vi "Test Get Data.vi"() -> ()   [LabVIEW 2014]
uses:
  FPGA/Rate.ctl
  <vilib>/FPGAPlugInAG/sbRIO-9636/niLvFpga_Open_sbRIO-9636.vi
  <vilib>/Utility/error.llb/Error Cluster From Error Code.vi
  <vilib>/rvi/errors/niLvFpgaAdjustHostInterfaceError.vi
  <vilib>/rvi/interface/common/niFpgaWaitOnOcc.vi
  <vilib>/FPGAPlugInAG/sbRIO-9636/niLvFpga_Close_sbRIO-9636.vi
  <vilib>/rvi/interface/nirviOpenFPGA/nirviOpenFPGA.xnode
  CRD/tFPGA Ref.ctl
  FPGA Bitfiles/FPGAServerwLRS.lvbitx
  <vilib>/rvi/interface/nirviReadWriteControl/nirviReadWriteControl.xnode
  <vilib>/rvi/interface/nirviMethod/nirviMethod.xnode
  <vilib>/rvi/interface/nirviCloseFPGA/nirviCloseFPGA.xnode
  CRD/tCRD.lvclass
  <vilib>/FPGAPlugInAG/sbRIO-9636/niLvFpga_ConfigureFifo_sbRIO-9636.vi
  <vilib>/rvi/errors/niLvFpgaMergeErrorWithErrorCode.vi
  NiFpgaLv.dll
  <vilib>/FPGAPlugInAG/sbRIO-9636/niLvFpga_StartFifo_sbRIO-9636.vi
  <vilib>/FPGAPlugInAG/sbRIO-9636/niLvFpga_StopFifo_sbRIO-9636.vi
  <vilib>/FPGAPlugInAG/sbRIO-9636/niLvFpga_ReadFifo_sbRIO-9636.vi
panel:
  in  "max":i32
  out "Elements Remaining":u32
  out "NewData":u16
  out "NumElements":u32
  out "DataLoop":bool
  in  "Stop Button":bool
  out "error out":errorcluster
  out "Data":i16[](array[numeric])
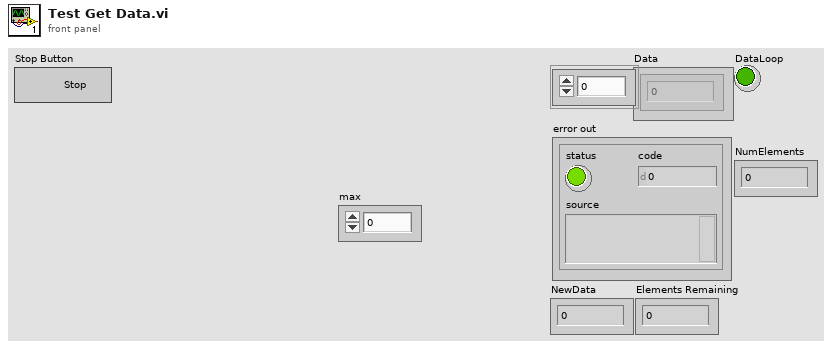
[diagram p1: front panel]
types:
  T1 = typedef "Rate.ctl" = u8
  T2 = typedef "tCRD.lvclass/tFPGA Ref.ctl" = refnum<k20>
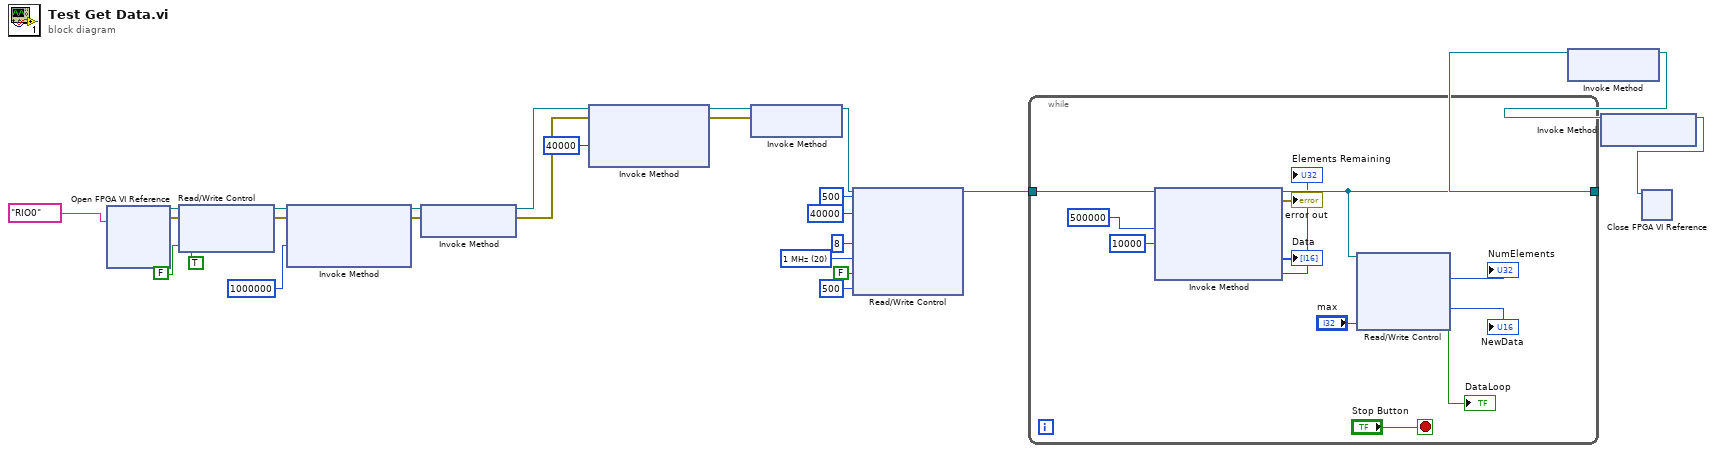
[diagram p0: block diagram]
diagram:
  w6 = T1 20 items=["1 MHz"=20, "2 MHz"=10, "2.5 MHz"=8, "5 MHz"=4, "10 MHz"=2, "20MHz"=1] ("Rate")
  n1 = xnode "Open FPGA VI Reference"("resource name"=tag "RIO0") -> ("FPGA VI Reference Out"=w25:T2, "error out"=w24:errorcluster)  [unwired: 1 in]
  n2 = xnode ("Read/Write Control")("FPGA VI Reference In"=w25, "error in"=w24, "Pause Digitizer"=TRUE, "Reverse?"=FALSE) -> ("FPGA VI Reference Out"=w19:T2, "error out"=w18:errorcluster)
  n3 = xnode "Invoke Method"("FPGA VI Reference In"=w19, "error in"=w18, "Requested Depth"=u32 1000000) -> ("FPGA VI Reference Out"=w23:T2, "error out"=w22:errorcluster)  [unwired: 1 out]
  n4 = xnode "Invoke Method"("FPGA VI Reference In"=w23, "error in"=w22) -> ("FPGA VI Reference Out"=w12:T2, "error out"=w17:errorcluster)
  n5 = xnode "Invoke Method"("FPGA VI Reference In"=w12, "error in"=w17, "Requested Depth"=u32 40000) -> ("FPGA VI Reference Out"=w16:T2, "error out"=w15:errorcluster)  [unwired: 1 out]
  n6 = xnode "Invoke Method"("FPGA VI Reference In"=w16, "error in"=w15) -> ("FPGA VI Reference Out"=w11:T2)  [unwired: 1 out]
  n7 = xnode "Read/Write Control"("FPGA VI Reference In"=w11, "Cylce (ticks)"=u32 40000, "Sample Time (us)"=u16 500, "Delay (us)"=u16 8, "Rate"=w6, "Pause Digitizer"=FALSE, "LaserOff (us)"=u32 500) -> ("FPGA VI Reference Out"=w4:T2)  [unwired: 1 in, 1 out]
  n8 = while {
    tunnel: w4 -> [w38]
    tunnel: [w32] -> w3
    stop <- "Stop Button" stop-if-true
    n9 = xnode "Invoke Method"("FPGA VI Reference In"=w38, "Number of Elements"=u32 500000, "Timeout (ms)"=10000) -> ("FPGA VI Reference Out"=w32:T2, "error out"=→"error out":errorcluster, "Data"=→"Data":i16[], "Elements Remaining"=→"Elements Remaining":u32)  [unwired: 1 in]
    n10 = xnode "Read/Write Control"("FPGA VI Reference In"=w32, "max"="max") -> ("NumElements"=→"NumElements":u32, "ShipLoop"=→"DataLoop":bool, "NewData"=→"NewData":u16)  [unwired: 1 in, 2 out]
  }
  n11 = xnode "Invoke Method"("FPGA VI Reference In"=w3) -> ("FPGA VI Reference Out"=w2:T2)  [unwired: 1 in, 1 out]
  n12 = xnode "Invoke Method"("FPGA VI Reference In"=w2) -> ("FPGA VI Reference Out"=w1:T2)  [unwired: 1 in, 1 out]
  n13 = xnode "Close FPGA VI Reference"("FPGA VI Reference In"=w1) -> ()  [unwired: 1 in, 1 out]
